vi "Test Initialized.vi"(8 "error in (no error)":errorcluster) -> (0 "error out":errorcluster, 3 "body":string)   [LabVIEW 2020, in "MCP Server tests.lvlib"]
uses:
  MCP Server tests.lvlib
  <vilib>/addons/_JKI Toolkits/Caraya/classes/Test/Test.lvclass
  <vilib>/addons/_JKI Toolkits/Caraya/classes/Assert/Assert.lvclass
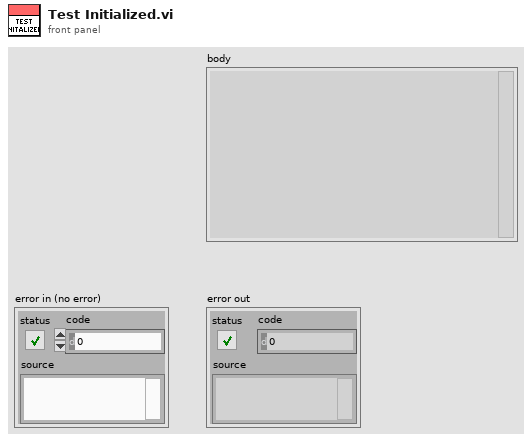
[diagram p1: front panel]
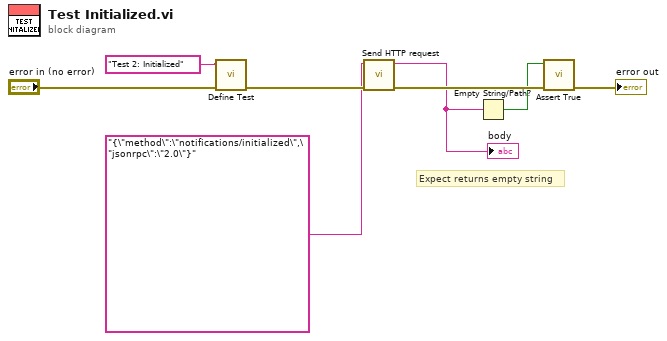
[diagram p0: block diagram]
diagram:
  # "Expect returns empty string"
  n1 = call <vilib>:"Define Test.vi"("error in (no error)"="error in (no error)", "Label (VI Title)"="Test 2: Initialized") -> ("error out"=w7:errorcluster)  [unwired: 8 in, 1 out]
  n2 = call "Send HTTP request.vi"("error in (no error)"=w7, "request"="{\"method\":\"notifications/initialized\",\"jsonrpc\":\"2.0\"}" ("buffer")) -> ("error out"=w8:errorcluster, "response"=w2:string)  [unwired: 7 in, 1 out]
  "body" <- w2
  n3 = Empty String/Path?(string/path=w2) -> (empty?=w1:bool)
  n4 = call <vilib>:"Assert True.vi"("error in (no error)"=w8, "True?"=w1) -> ("error out"=→"error out":errorcluster)  [unwired: 8 in, 1 out]
